vi "main.vi"() -> ()   [LabVIEW 2016]
uses:
  <instrlib>/Lake Shore 425/Public/Data/Field Data (Single Reading).vi
  <instrlib>/Agilent 3446X Series/Public/Data/Read (Single Point).vi
  <instrlib>/Lake Shore 425/Lake Shore 425.lvlib
  <instrlib>/Lake Shore Cryotronics 218/Lake Shore Cryotronics 218.lvlib
  <instrlib>/Agilent 3446X Series/Agilent 3446X Series.lvlib
panel:
  in  "milliseconds to wait":u32
  in  "Stop Button":bool
  out "Probe 3 Type":u16(ring) caption="Probe Type"
  out "Probe 2 Type":u16(ring) caption="Probe Type"
  in  "Y-Axis of Graph":u16(ring) items=["Time", "X-Position", "Y-Position", "Z-Position", "Gaussmeter 1", "Gaussmeter 2", "Gaussmeter 3", "Multimeter", "Temp. Sensor 1", "Temp. Sensor 2", "Temp. Sensor 3", "Temp. Sensor 4", "Temp. Sensor 5", "Temp. Sensor 6", "Temp. Sensor 7", "Temp. Sensor 8"]
  in  "X-Axis of Graph":u16(ring) items=["Time", "X-Position", "Y-Position", "Z-Position", "Gaussmeter 1", "Gaussmeter 2", "Gaussmeter 3", "Multimeter", "Temp. Sensor 1", "Temp. Sensor 2", "Temp. Sensor 3", "Temp. Sensor 4", "Temp. Sensor 5", "Temp. Sensor 6", "Temp. Sensor 7", "Temp. Sensor 8"]
  out "XY Graph":cluster{"X":dbl, "Y":dbl}[](graph)
  out "Temperature Monitor Chart":dbl[](graph)
  out "Multimeter Chart":dbl(graph)
  out "Gaussmeter 3 Chart":dbl(graph)
  out "Gaussmeter 2 Chart":dbl(graph)
  out "Gaussmeter 1 Chart":dbl(graph)
  in  "z Multimeter":dbl caption="z"
  in  "y Multimeter":dbl caption="y"
  in  "x Multimeter":dbl caption="x"
  in  "z Gaussmeter 3":dbl caption="z"
  in  "y Gaussmeter 3":dbl caption="y"
  in  "x Gaussmeter 3":dbl caption="x"
  in  "z Gaussmeter 2":dbl caption="z"
  in  "y Gaussmeter 2":dbl caption="y"
  in  "x Gaussmeter 2":dbl caption="x"
  in  "z Gaussmeter 1":dbl caption="z"
  in  "y Gaussmeter 1":dbl caption="y"
  in  "x Gaussmeter 1":dbl caption="x"
  in  "Temp. Sensors Moving":bool[](array[boolean])
  in  "Multimeter Moving":bool
  in  "Gaussmeter 3 Moving":bool
  in  "Gaussmeter 2 Moving":bool
  in  "Gaussmeter 1 Moving":bool
  out "Field Map File Name":string
  in  "Field Map File Path":path
  in  "Field Map":bool
  in  "Measurement Type":u16(ring) items=["Current (3 A)", "Current (10 A)", "Shunt Voltage (50A - 50mV)"]
  in  "Sensor 8":bool
  in  "Sensor 7":bool
  in  "Sensor 6":bool
  in  "Sensor 5":bool
  in  "Sensor 4":bool
  in  "Sensor 3":bool
  in  "Sensor 2":bool
  in  "Sensor 1":bool
  in  "Probe 3 Zero":bool
  in  "Probe 2 Zero":bool
  in  "Probe 1 Zero":bool
  out "Time [s]":dbl
  out "Duration [s]":dbl
  in  "Seconds":dbl
  in  "Minutes":dbl
  in  "Hours":dbl
  out "Temp. Monitor Status":bool caption="Working"
  in  "On/Off Temp. Monitor":bool
  in  "VISA Temp. Monitor":refnum<visa-resource-name>
  out "Multimeter Status":bool caption="Working"
  in  "On/Off Multimeter":bool
  in  "VISA Multimeter":refnum<visa-resource-name>
  out "Probe 3 Status":bool caption="Working"
  out "Probe 3 Field Comp.":bool caption="Field\nComp."
  out "Probe 3 Serial Number":string caption="Probe Serial Number"
  out "Probe 3 Sensitivity":dbl caption="Probe Sensitivity"
  in  "On/Off Gaussmeter 3":bool
  in  "VISA Gaussmeter 3":refnum<visa-resource-name>
  out "Probe 2 Status":bool caption="Working"
  out "Probe 2 Field Comp.":bool caption="Field\nComp."
  out "Probe 2 Serial Number":string caption="Probe Serial Number"
  out "Probe 2 Sensitivity":dbl caption="Probe Sensitivity"
  in  "On/Off Gaussmeter 2":bool
  in  "VISA Gaussmeter 2":refnum<visa-resource-name>
  out "Probe 1 Status":bool caption="Working"
  out "Probe 1 Field Comp.":bool caption="Field\nComp."
  out "Probe 1 Serial Number":string caption="Probe Serial Number"
  out "Probe 1 Sensitivity":dbl caption="Probe Sensitivity"
  out "Probe 1 Type":u16(ring) caption="Probe Type"
  in  "On/Off Gaussmeter 1":bool
  in  "VISA Gaussmeter 1":refnum<visa-resource-name>
  out "Output File Name":string
  out "Output File Path":path
  in  "Output Folder Path":path
  # "Gaussmeter 1"
  # "Gaussmeter 2"
  # "Gaussmeter 3"
  # "Multimeter"
  # "Temperature Monitor"
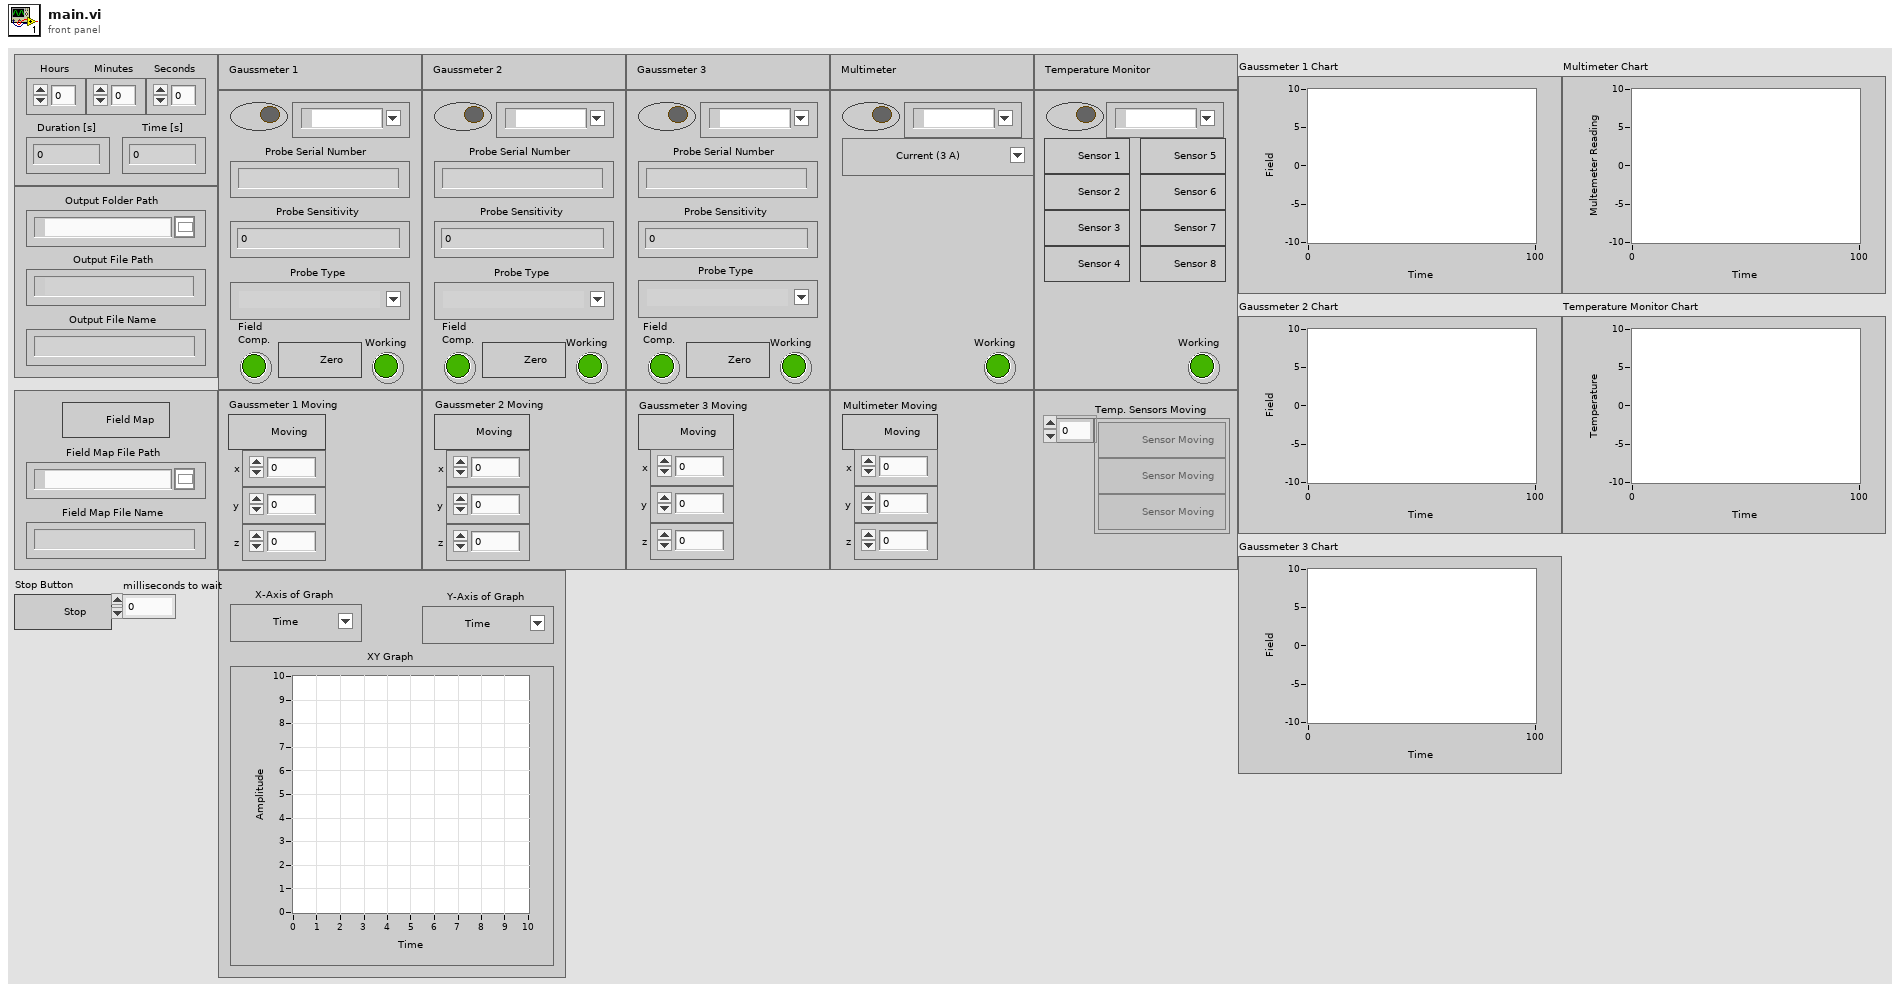
[diagram p1: front panel]
types:
  T1 = enum16{"open", "replace", "create", "open or create", "replace or create", "replace or create with confirmation"}
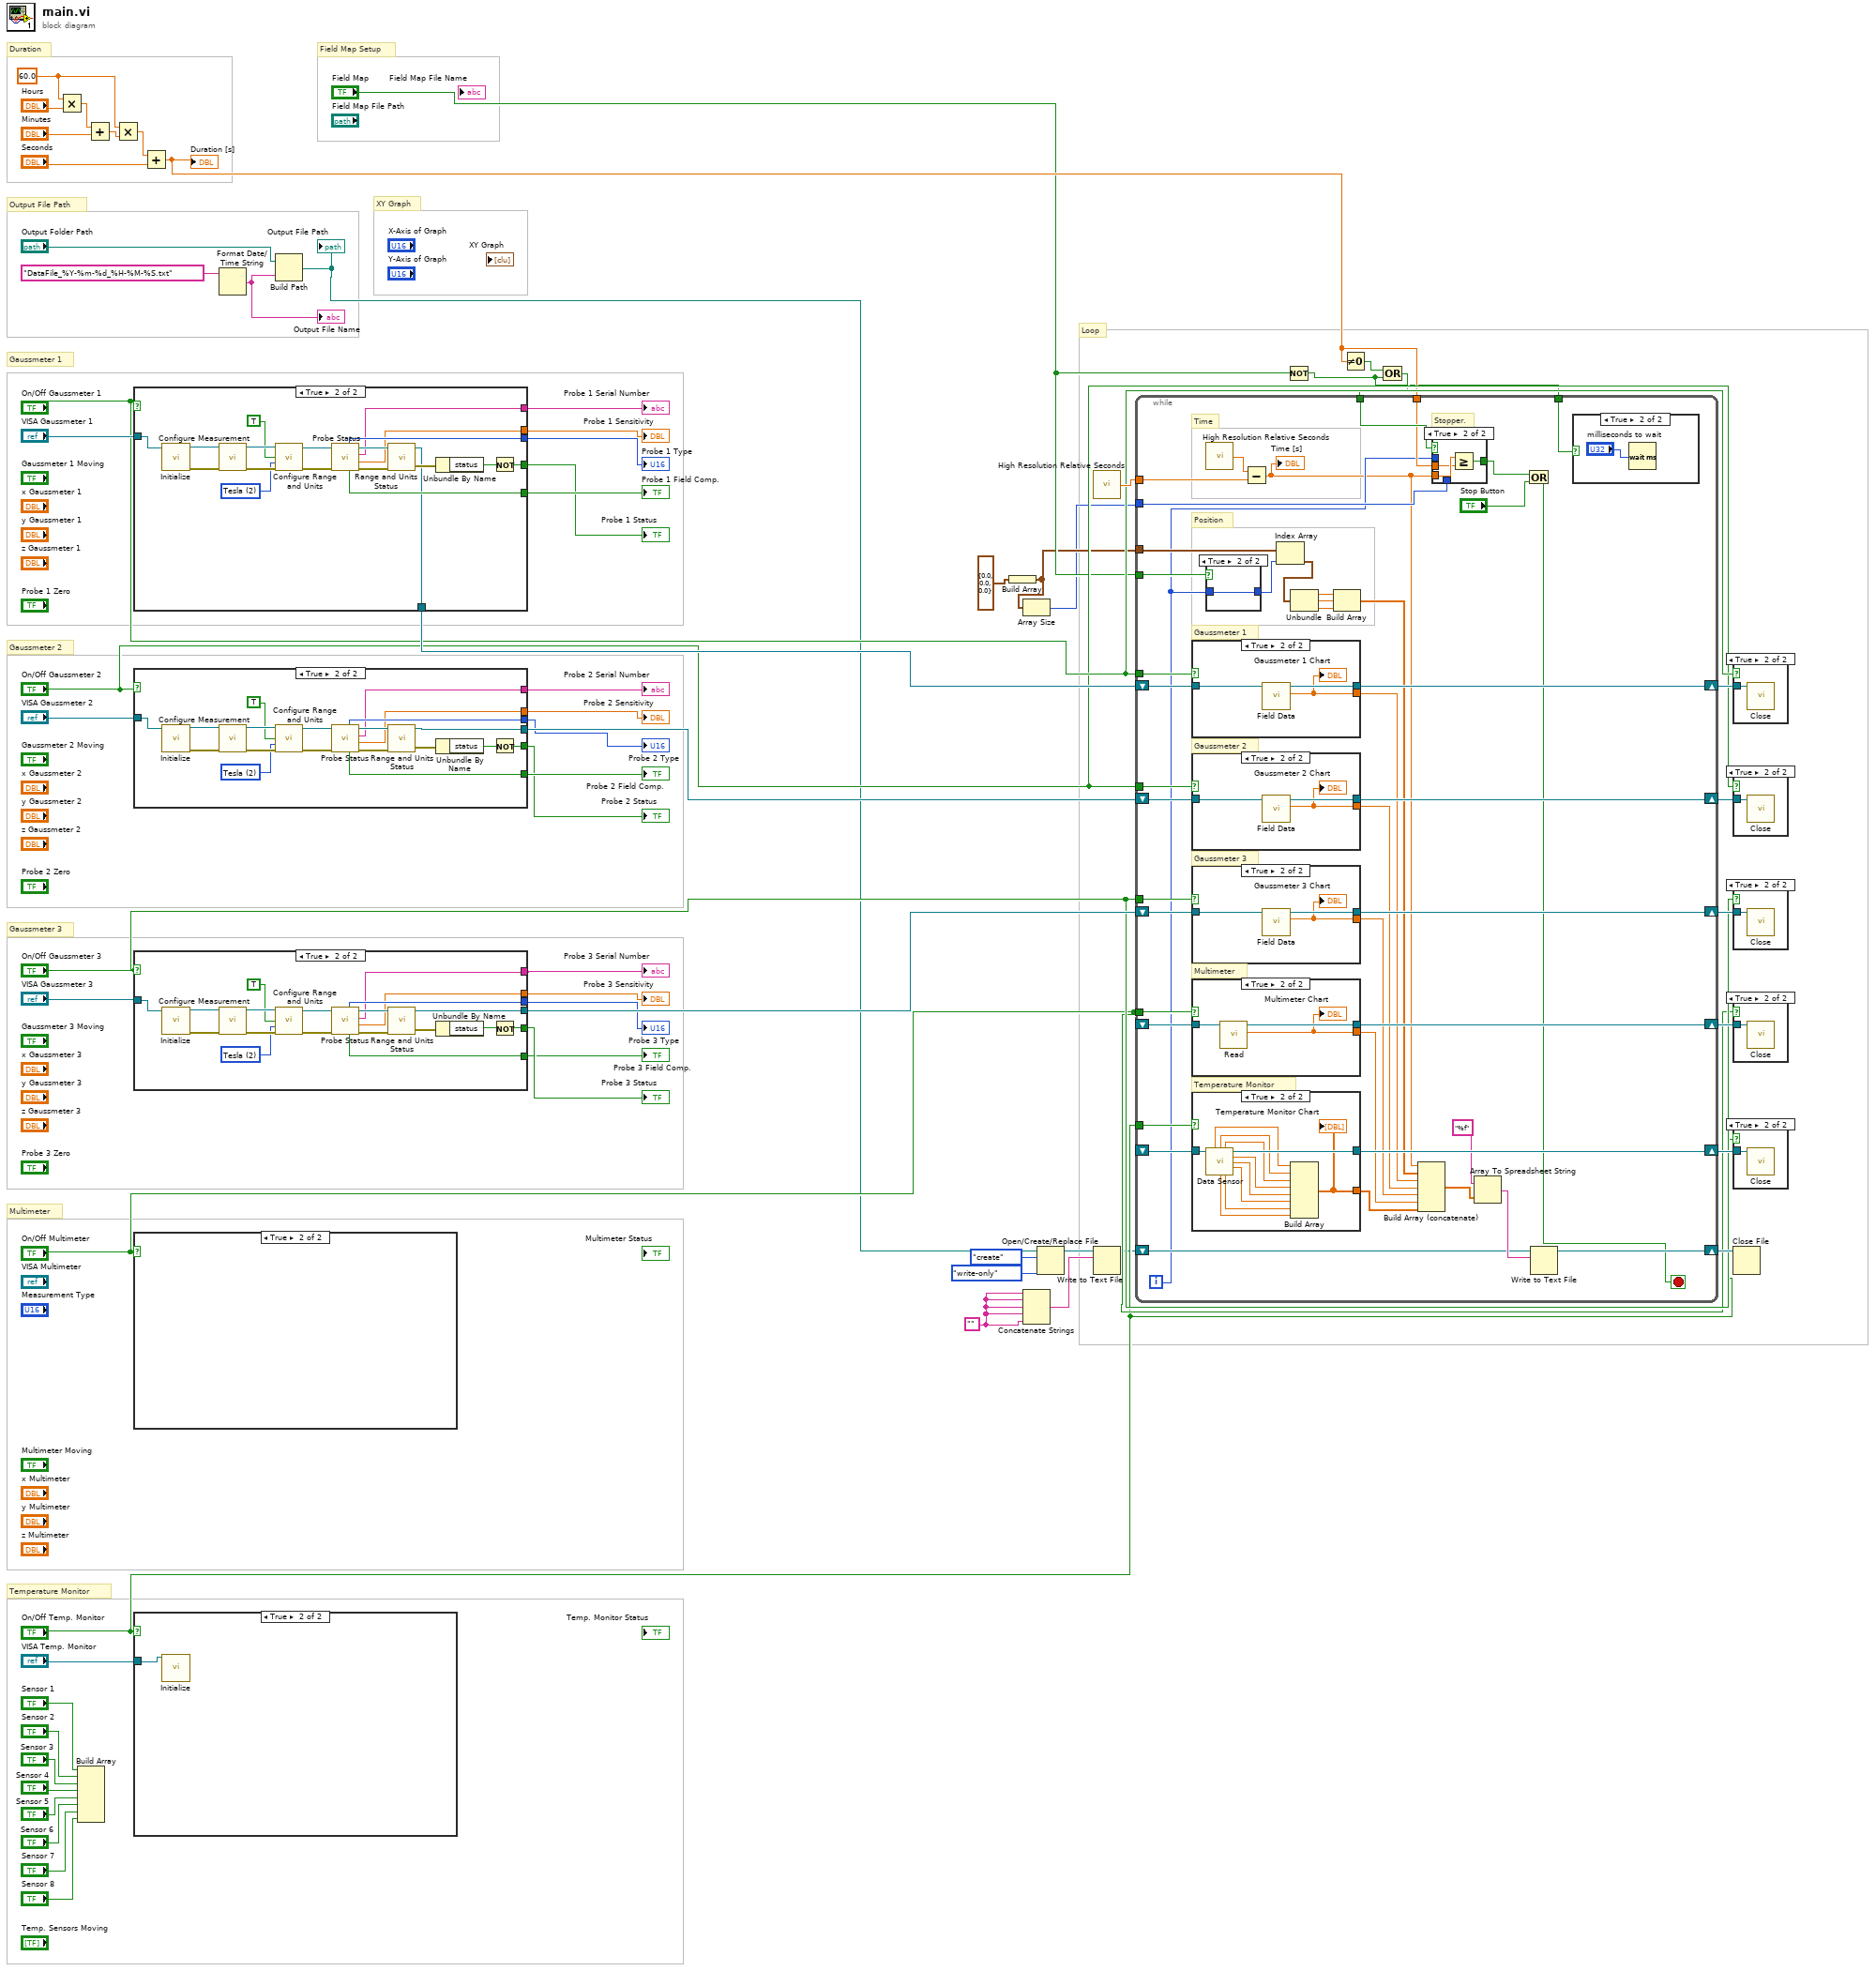
[diagram p0: block diagram]
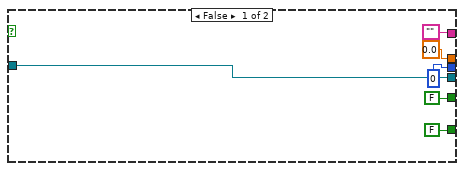
[diagram p2: hidden frame]
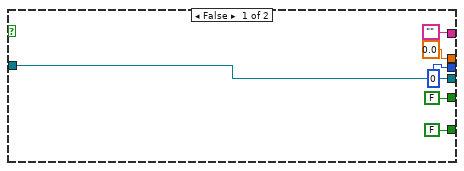
[diagram p3: hidden frame]
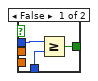
[diagram p10: hidden frame]
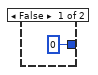
[diagram p11: hidden frame]
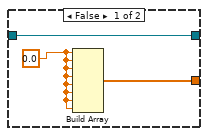
[diagram p12: hidden frame]
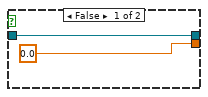
[diagram p13: hidden frame]
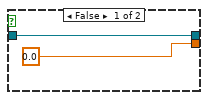
[diagram p14: hidden frame]
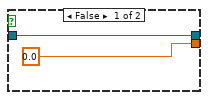
[diagram p15: hidden frame]
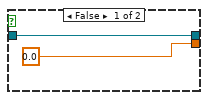
[diagram p16: hidden frame]
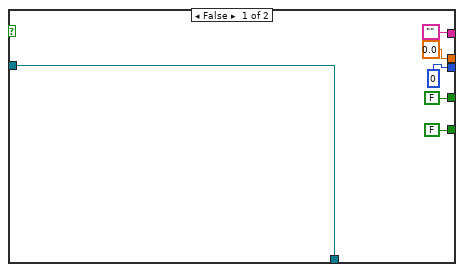
[diagram p19: hidden frame]
diagram:
  w5 = ""
  w63 = 60.0
  # "Loop"
  # "XY Graph"
  # "Field Map Setup"
  # "Temperature Monitor"
  # "Multimeter"
  # "Gaussmeter 3"
  # "Gaussmeter 2"
  # "Gaussmeter 1"
  # "Output File Path"
  # "Duration"
  n1 = Multiply(x=w63, y="Hours") -> (x*y=w65:dbl)
  n2 = Build Array("Sensor 1", "Sensor 2", "Sensor 3", "Sensor 4", "Sensor 5", "Sensor 6", "Sensor 7", "Sensor 8") -> ()  [unwired: 1 out]
  n3 = Add(x=w65, y="Minutes") -> (x+y=w64:dbl)
  n4 = Multiply(x=w63, y=w64) -> (x*y=w62:dbl)
  n5 = case shown="True" "On/Off Gaussmeter 1" {
    tunnel: "VISA Gaussmeter 1" -> [w68 w92]
    tunnel: [u16 0 w82] -> w58
    tunnel: ["" w81] -> w57
    tunnel: [0.0 w80] -> w56
    tunnel: [FALSE w78] -> w55
    tunnel: [FALSE w75] -> w54
    tunnel: [w68 w74] -> w36
    frame False {
    }
    frame True {
      w86 = u16 2 items=["Gauss"=1, "Tesla"=2, "Oersted"=3, "Amp/meter"=4] ("Field Units (1:Gauss)")
      n6 = call <instrlib>:"Initialize.vi"("VISA resource name"=w92) -> ("error out"=w90:errorcluster, "VISA resource name out"=w91:refnum<visa-resource-name>)  [unwired: 9 in]
      n7 = call <instrlib>:"Configure Measurement.vi"("VISA resource name"=w91, "error in (no error)"=w90) -> ("VISA resource name out"=w89:refnum<visa-resource-name>, "error out"=w87:errorcluster)  [unwired: 12 in]
      n8 = call <instrlib>:"Configure Range and Units.vi"("VISA resource name"=w89, "Auto Range (F: Off)"=TRUE, "Field Units (1:Gauss)"=w86, "error in (no error)"=w87) -> ("VISA resource name out"=w85:refnum<visa-resource-name>, "error out"=w79:errorcluster)  [unwired: 10 in]
      n9 = call <instrlib>:"Probe Status.vi"("error in (no error)"=w79, "VISA resource name"=w85) -> ("error out"=w83:errorcluster, "Probe Sensitivity"=w80:dbl, "Probe Serial Number"=w81:string, "VISA resource name out"=w84:refnum<visa-resource-name>, "Probe Field \nCompensation On"=w78:bool, "Probe Type"=w82:u16)  [unwired: 4 in]
      n10 = call <instrlib>:"Range and Units Status.vi"("error in (no error)"=w83, "VISA resource name"=w84) -> ("error out"=w77:errorcluster, "VISA resource name out"=w74:refnum<visa-resource-name>)  [unwired: 5 in, 3 out]
      n11 = Unbundle By Name(w77) -> ("status"=w76:bool)
      n12 = Not(x=w76) -> (.not. x?=w75:bool)
    }
  }
  "Probe 1 Type" <- w58
  "Probe 1 Sensitivity" <- w56
  "Probe 1 Serial Number" <- w57
  "Probe 1 Field Comp." <- w55
  "Probe 1 Status" <- w54
  n13 = case shown="True" "On/Off Gaussmeter 2" {
    tunnel: "VISA Gaussmeter 2" -> [w93 w117]
    tunnel: [u16 0 w107] -> w29
    tunnel: ["" w106] -> w31
    tunnel: [0.0 w105] -> w30
    tunnel: [FALSE w103] -> w25
    tunnel: [FALSE w100] -> w24
    tunnel: [w93 w99] -> w35
    frame False {
    }
    frame True {
      w111 = u16 2 items=["Gauss"=1, "Tesla"=2, "Oersted"=3, "Amp/meter"=4] ("Field Units (1:Gauss)")
      n14 = call <instrlib>:"Initialize.vi"("VISA resource name"=w117) -> ("error out"=w115:errorcluster, "VISA resource name out"=w116:refnum<visa-resource-name>)  [unwired: 9 in]
      n15 = call <instrlib>:"Configure Measurement.vi"("VISA resource name"=w116, "error in (no error)"=w115) -> ("VISA resource name out"=w114:refnum<visa-resource-name>, "error out"=w112:errorcluster)  [unwired: 12 in]
      n16 = call <instrlib>:"Configure Range and Units.vi"("VISA resource name"=w114, "Auto Range (F: Off)"=TRUE, "Field Units (1:Gauss)"=w111, "error in (no error)"=w112) -> ("VISA resource name out"=w110:refnum<visa-resource-name>, "error out"=w104:errorcluster)  [unwired: 10 in]
      n17 = call <instrlib>:"Probe Status.vi"("error in (no error)"=w104, "VISA resource name"=w110) -> ("error out"=w108:errorcluster, "Probe Sensitivity"=w105:dbl, "Probe Serial Number"=w106:string, "VISA resource name out"=w109:refnum<visa-resource-name>, "Probe Field \nCompensation On"=w103:bool, "Probe Type"=w107:u16)  [unwired: 4 in]
      n18 = call <instrlib>:"Range and Units Status.vi"("error in (no error)"=w108, "VISA resource name"=w109) -> ("error out"=w102:errorcluster, "VISA resource name out"=w99:refnum<visa-resource-name>)  [unwired: 5 in, 3 out]
      n19 = Unbundle By Name(w102) -> ("status"=w101:bool)
      n20 = Not(x=w101) -> (.not. x?=w100:bool)
    }
  }
  "Probe 2 Status" <- w24
  "Probe 2 Field Comp." <- w25
  "Probe 2 Serial Number" <- w31
  "Probe 2 Sensitivity" <- w30
  "Probe 2 Type" <- w29
  n21 = case shown="True" "On/Off Gaussmeter 3" {
    tunnel: "VISA Gaussmeter 3" -> [w118 w142]
    tunnel: [u16 0 w132] -> w28
    tunnel: ["" w131] -> w26
    tunnel: [0.0 w130] -> w27
    tunnel: [FALSE w128] -> w22
    tunnel: [FALSE w125] -> w23
    tunnel: [w118 w124] -> w34
    frame False {
    }
    frame True {
      w136 = u16 2 items=["Gauss"=1, "Tesla"=2, "Oersted"=3, "Amp/meter"=4] ("Field Units (1:Gauss)")
      n22 = call <instrlib>:"Initialize.vi"("VISA resource name"=w142) -> ("error out"=w140:errorcluster, "VISA resource name out"=w141:refnum<visa-resource-name>)  [unwired: 9 in]
      n23 = call <instrlib>:"Configure Measurement.vi"("VISA resource name"=w141, "error in (no error)"=w140) -> ("VISA resource name out"=w139:refnum<visa-resource-name>, "error out"=w137:errorcluster)  [unwired: 12 in]
      n24 = call <instrlib>:"Configure Range and Units.vi"("VISA resource name"=w139, "Auto Range (F: Off)"=TRUE, "Field Units (1:Gauss)"=w136, "error in (no error)"=w137) -> ("VISA resource name out"=w135:refnum<visa-resource-name>, "error out"=w129:errorcluster)  [unwired: 10 in]
      n25 = call <instrlib>:"Probe Status.vi"("error in (no error)"=w129, "VISA resource name"=w135) -> ("error out"=w133:errorcluster, "Probe Sensitivity"=w130:dbl, "Probe Serial Number"=w131:string, "VISA resource name out"=w134:refnum<visa-resource-name>, "Probe Field \nCompensation On"=w128:bool, "Probe Type"=w132:u16)  [unwired: 4 in]
      n26 = call <instrlib>:"Range and Units Status.vi"("error in (no error)"=w133, "VISA resource name"=w134) -> ("error out"=w127:errorcluster, "VISA resource name out"=w124:refnum<visa-resource-name>)  [unwired: 5 in, 3 out]
      n27 = Unbundle By Name(w127) -> ("status"=w126:bool)
      n28 = Not(x=w126) -> (.not. x?=w125:bool)
    }
  }
  "Probe 3 Status" <- w23
  "Probe 3 Field Comp." <- w22
  "Probe 3 Serial Number" <- w26
  "Probe 3 Sensitivity" <- w27
  "Probe 3 Type" <- w28
  n29 = case shown="True" "On/Off Multimeter" {
    frame False {
    }
    frame True {
    }
  }
  n30 = case shown="True" "On/Off Temp. Monitor" {
    tunnel: "VISA Temp. Monitor" -> [_ w143]
    frame False {
    }
    frame True {
      n31 = call <instrlib>:"Initialize.vi"("VISA resource name"=w143) -> ()  [unwired: 13 in, 2 out]
    }
  }
  n32 = Add(x=w62, y="Seconds") -> (x+y=w16:dbl)
  "Duration [s]" <- w16
  n33 = Format Date/Time String(time format string (%c)="DataFile_%Y-%m-%d_%H-%M-%S.txt") -> (date/time string=w3:string)  [unwired: 2 in]
  "Output File Name" <- w3
  n34 = Build Path(base path="Output Folder Path", name or relative path=w3) -> (appended path=w4:path)
  "Output File Path" <- w4
  n35 = Build Array(cluster{dbl, dbl, dbl} {0.0, 0.0, 0.0}) -> (w12:cluster{dbl, dbl, dbl}[])
  n36 = Array Size(array=w12) -> (size(s)=w11:i32)
  n37 = Concatenate Strings(w5, w5, w5, w5, w5) -> (w6:string)
  n38 = Open/Create/Replace File(file path (use dialog)=w4, operation (0:open)=T1."create", access (0:read/write)=enum16{"read/write", "read-only", "write-only"}."write-only") -> (refnum out=w9:refnum<file>)  [unwired: 3 in, 2 out]
  n39 = call <vilib>:"High Resolution Relative Seconds.vi"() -> ("relative seconds"=w37:dbl)
  n40 = Write to Text File(file (use dialog)=w9, text=w6) -> (refnum out=w10:refnum<file>)  [unwired: 2 in, 2 out]
  n41 = Not(x="Field Map") -> (.not. x?=w1:bool)
  n42 = Not Equal To 0?(x=w16) -> (x != 0?=w15:bool)
  n43 = Or(x=w15, y=w1) -> (x .or. y?=w14:bool)
  n44 = while {
    tunnel: "On/Off Temp. Monitor" -> [w172]
    tunnel: "On/Off Multimeter" -> [w171]
    tunnel: "On/Off Gaussmeter 3" -> [w170]
    tunnel: "On/Off Gaussmeter 1" -> [w169]
    shift-right: [w178] -> w38
    shift-left: w36 -> [w187]
    shift-right: [w179] -> w39
    shift-left: w35 -> [w186]
    shift-right: [w180] -> w40
    shift-left: w34 -> [w185]
    shift-right: [w181] -> w41
    shift-left: _ -> [w184]
    shift-right: [w182] -> w42
    shift-left: _ -> [w183]
    tunnel: "Field Map" -> [w167]
    tunnel: w37 -> [w166]
    tunnel: w12 -> [w161]
    shift-right: [w155] -> w43
    shift-left: w10 -> [w156]
    tunnel: "On/Off Gaussmeter 2" -> [w154]
    tunnel: w14 -> [w152]
    tunnel: w16 -> [w151]
    tunnel: w11 -> [w150]
    tunnel: w1 -> [w144]
    i -> [w149]
    stop <- w147 stop-if-true
    # "Stopper."
    # "Position"
    # "Time"
    # "Temperature Monitor"
    # "Multimeter"
    # "Gaussmeter 3"
    # "Gaussmeter 2"
    # "Gaussmeter 1"
    n45 = case shown="True" w169 {
      tunnel: w187 -> [w227 w230]
      tunnel: [w227 w229] -> w178
      tunnel: [0.0 w228] -> w173
      frame False {
      }
      frame True {
        n46 = call-poly <instrlib>:"Field Data.vi"("VISA resource name"=w230) -> ("Field Reading"=w228:dbl, "VISA resource name out"=w229:refnum<visa-resource-name>)  [unwired: 8 in, 1 out]
        "Gaussmeter 1 Chart" <- w228
      }
    }
    n47 = case shown="True" w154 {
      tunnel: w186 -> [w222 w225]
      tunnel: [w222 w224] -> w179
      tunnel: [0.0 w223] -> w175
      frame False {
      }
      frame True {
        n48 = call-poly <instrlib>:"Field Data.vi"("VISA resource name"=w225) -> ("Field Reading"=w223:dbl, "VISA resource name out"=w224:refnum<visa-resource-name>)  [unwired: 8 in, 1 out]
        "Gaussmeter 2 Chart" <- w223
      }
    }
    n49 = case shown="True" w170 {
      tunnel: w185 -> [w217 w220]
      tunnel: [w217 w219] -> w180
      tunnel: [0.0 w218] -> w174
      frame False {
      }
      frame True {
        n50 = call-poly <instrlib>:"Field Data.vi"("VISA resource name"=w220) -> ("Field Reading"=w218:dbl, "VISA resource name out"=w219:refnum<visa-resource-name>)  [unwired: 8 in, 1 out]
        "Gaussmeter 3 Chart" <- w218
      }
    }
    n51 = case shown="True" w171 {
      tunnel: w184 -> [w212 w215]
      tunnel: [w212 w214] -> w181
      tunnel: [0.0 w213] -> w176
      frame False {
      }
      frame True {
        n52 = call-poly <instrlib>:"Read.vi"("VISA resource name"=w215) -> ("Measurement"=w213:dbl, "VISA resource name out"=w214:refnum<visa-resource-name>)  [unwired: 8 in, 1 out]
        "Multimeter Chart" <- w213
      }
    }
    n53 = case shown="True" w172 {
      tunnel: w183 -> [w199 w210]
      tunnel: [w199 w209] -> w182
      tunnel: [w198 w200] -> w177
      frame False {
        w197 = 0.0
        n54 = Build Array(w197, w197, w197, w197, w197, w197, w197, w197) -> (w198:dbl[])
      }
      frame True {
        n55 = call <instrlib>:"Data Sensor.vi"("VISA resource name"=w210) -> ("Input 1"=w203:dbl, "Input 2"=w204:dbl, "Input 3"=w205:dbl, "VISA resource name out"=w209:refnum<visa-resource-name>, "Input 4"=w201:dbl, "Input 5"=w202:dbl, "Input 6"=w208:dbl, "Input 8"=w206:dbl, "Input 7"=w207:dbl)  [unwired: 5 in, 1 out]
        n56 = Build Array(w203, w204, w205, w201, w202, w208, w207, w206) -> (w200:dbl[])
        "Temperature Monitor Chart" <- w200
      }
    }
    n57 = call <vilib>:"High Resolution Relative Seconds.vi"() -> ("relative seconds"=w168:dbl)
    n58 = case shown="True" w167 {
      tunnel: w149 -> [_ w196]
      tunnel: [0 w196] -> w162
      frame False {
      }
      frame True {
      }
    }
    n59 = Subtract(x=w168, y=w166) -> (x-y=w145:dbl)
    "Time [s]" <- w145
    n60 = Index Array(array=w161, index=w162) -> (element=w159:cluster{dbl, dbl, dbl})
    n61 = Unbundle(w159) -> (w163:dbl, w164:dbl, w165:dbl)
    n62 = Build Array(w163, w164, w165) -> (w160:dbl[])
    n63 = Build Array (concatenate)(w145, w160, w173, w175, w174, w176, w177) -> (w158:dbl[])
    n64 = case shown="True" w152 {
      tunnel: w145 -> [_ w194]
      tunnel: w151 -> [_ w193]
      tunnel: [w191 w192] -> w148
      tunnel: w150 -> [w189 _]
      tunnel: w149 -> [w190 _]
      frame False {
        n65 = Greater Or Equal?(x=w190, y=w189) -> (x >= y?=w191:bool)
      }
      frame True {
        n66 = Greater Or Equal?(x=w194, y=w193) -> (x >= y?=w192:bool)
      }
    }
    n67 = Array To Spreadsheet String(array=w158, 3:"%f" ("format string")) -> (spreadsheet string=w157:string)  [unwired: 1 in]
    n68 = Or(x=w148, y="Stop Button") -> (x .or. y?=w147:bool)
    n69 = Write to Text File(file (use dialog)=w156, text=w157) -> (refnum out=w155:refnum<file>)  [unwired: 2 in, 2 out]
    n70 = case shown="True" w144 {
      frame False {
      }
      frame True {
        n71 = Wait (ms)(milliseconds to wait="milliseconds to wait") -> ()  [unwired: 1 out]
      }
    }
  }
  n72 = case shown="True" "On/Off Gaussmeter 1" {
    tunnel: w38 -> [_ w231]
    frame False {
    }
    frame True {
      n73 = call <instrlib>:"Close.vi"("VISA resource name"=w231) -> ()  [unwired: 10 in, 1 out]
    }
  }
  n74 = case shown="True" "On/Off Gaussmeter 2" {
    tunnel: w39 -> [_ w232]
    frame False {
    }
    frame True {
      n75 = call <instrlib>:"Close.vi"("VISA resource name"=w232) -> ()  [unwired: 10 in, 1 out]
    }
  }
  n76 = case shown="True" "On/Off Gaussmeter 3" {
    tunnel: w40 -> [_ w233]
    frame False {
    }
    frame True {
      n77 = call <instrlib>:"Close.vi"("VISA resource name"=w233) -> ()  [unwired: 10 in, 1 out]
    }
  }
  n78 = case shown="True" "On/Off Multimeter" {
    tunnel: w41 -> [_ w234]
    frame False {
    }
    frame True {
      n79 = call <instrlib>:"Close.vi"("VISA resource name"=w234) -> ()  [unwired: 10 in, 1 out]
    }
  }
  n80 = case shown="True" "On/Off Temp. Monitor" {
    tunnel: w42 -> [_ w235]
    frame False {
    }
    frame True {
      n81 = call <instrlib>:"Close.vi"("VISA resource name"=w235) -> ()  [unwired: 14 in, 1 out]
    }
  }
  n82 = Close File(refnum=w43) -> ()  [unwired: 1 in, 2 out]
